vi "OA_SKit_scale to EU(new).vi"(4 "channel information":T2 {"sensor sensitivity (mV/EU)" format="%.2f"; "offset" format="%.2f"; "multiplier" format="%.2f"}, 7 "measured data":dbl[](array[numeric]) format="%.2f") -> (1 "unit lable":string, 2 "scaled data [EU]":dbl[](array[numeric]) format="%.2f", 3 "channel name":string)   [LabVIEW 2017]
uses:
  <vilib>/Analysis/NI_AALBase.lvlib
panel:
  in  "engineering units":T1(ring)
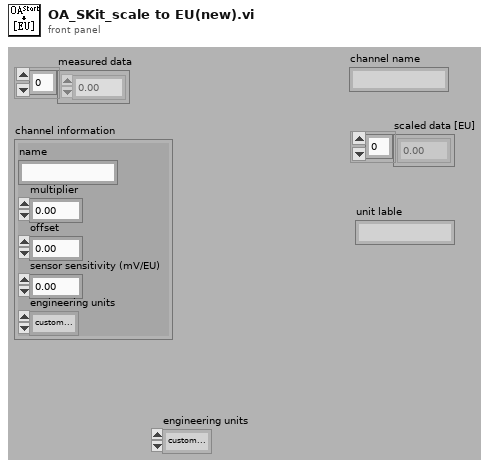
[diagram p1: front panel]
types:
  T1 = enum16{"custom...", "V", "Pa", "g", "m/s^2", "m/s", "m", "in/s^2", "in/s", "in"}
  T2 = cluster{"name":string, "multiplier":sgl, "offset":sgl, "sensor sensitivity (mV/EU)":dbl, "engineering units":enum16{"custom...", "V", "Pa", "g", "m/s^2", "m/s", "m", "in/s^2", "in/s", "in"}}
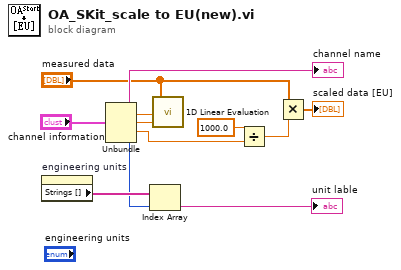
[diagram p0: block diagram]
diagram:
  n1 = property on="engineering units" class="Enum (strict)"() -> ("Strings []"=w8:string[])  [unwired: 2 in, 2 out]
  n2 = Unbundle("channel information") -> ("name"=→"channel name":string, "multiplier"=w11:sgl, "offset"=w10:sgl, "sensor sensitivity (mV/EU)"=w5:dbl, "engineering units"=w7:T1)
  n3 = Index Array(array=w8, index=w7) -> (element=→"unit lable":string)
  n4 = call <vilib>:"1D Linear Evaluation.vi"("offset"=w10, "scale"=w11, "X"="measured data") -> ()  [unwired: 2 out]
  n5 = Divide(x=1000.0, y=w5) -> (x/y=w4:dbl)
  n6 = Multiply(x="measured data", y=w4) -> (x*y=→"scaled data [EU]":dbl[])
